vi "S2C_ExeScriptBreakPt.vi"(8 "Error In":errorcluster, 11 "Row":i32) -> (0 "Error Out":errorcluster)   [LabVIEW 2015]
doc: "Toggles the breakpoint symbol, for the selected line, on the executable script table"
uses:
  Globals/S2C_Globals.vi
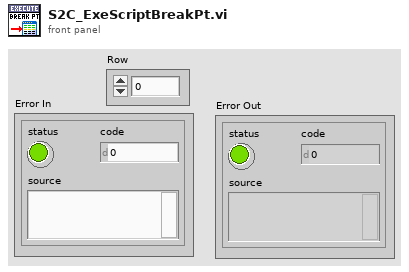
[diagram p1: front panel]
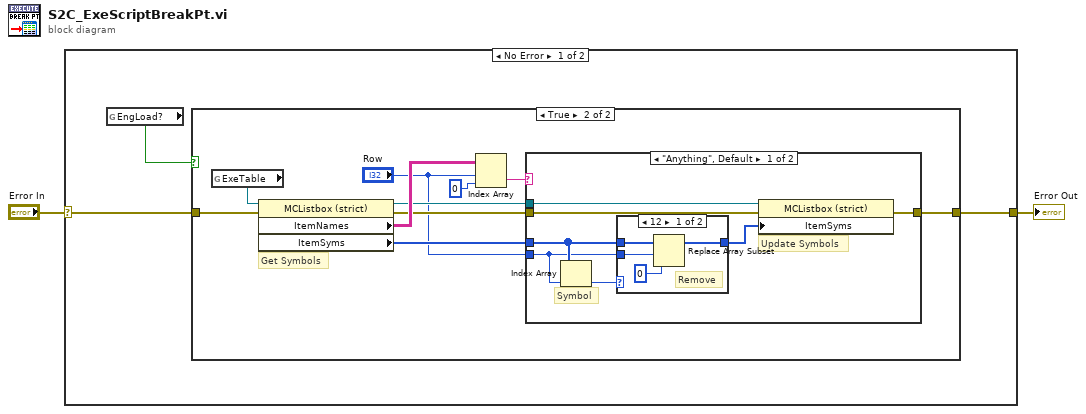
[diagram p0: block diagram]
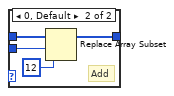
[diagram p3: hidden frame]
diagram:
  n1 = case shown="No Error" "Error In" {
    selector: "Error In" -> [w5 w33]
    tunnel: [w4 w33] -> w1
    frame No Error {
      n2 = global read "S2C_Globals.vi" "EngLoad?"() -> (w3:bool)
      n3 = case shown="True" w3 {
        tunnel: w5 -> [w6 w16]
        tunnel: [w6 w8] -> w4
        frame False {
          # "Breakpoints are only active for engineering loads"
        }
        frame True {
          # "Get Symbols"
          n4 = global read "S2C_Globals.vi" "ExeTable"() -> (w15:refnum<vi>)
          n5 = property class="MCListbox (strict)"(reference=w15, error in=w16) -> (reference out=w10:refnum<vi>, error out=w11:errorcluster, "ItemNames"=w14:string[][], "ItemSyms"=w9:i32[])
          n6 = Index Array(array=w14, index (row)="Row", index (col)=0 ("disabled index (col)")) -> (element=w12:string)
          n7 = case shown="\"Anything\", Default" w12 {
            tunnel: w11 -> [w20 w32]
            tunnel: w10 -> [w18 _]
            tunnel: w9 -> [w22 _]
            tunnel: [w17 w32] -> w8
            tunnel: "Row" -> [w21 _]
            frame "Anything", Default {
              # "Symbol"
              # "Update Symbols"
              n8 = Index Array(array=w22, index=w21) -> (element=w23:i32)
              n9 = case shown="12" w23 {
                tunnel: w22 -> [w27 w31]
                tunnel: w21 -> [w26 w30]
                tunnel: [w24 w28] -> w19
                frame 12 {
                  # "Remove"
                  n10 = Replace Array Subset(array=w27, new element=0, index=w26) -> (w24:i32[])
                }
                frame 0, Default {
                  # "Add"
                  n11 = Replace Array Subset(array=w31, new element=12, index=w30) -> (w28:i32[])
                }
              }
              n12 = property class="MCListbox (strict)"(reference=w18, error in=w20, "ItemSyms"=w19) -> (error out=w17:errorcluster)  [unwired: 1 out]
            }
            frame "" {
              # "Ignore if row blank"
            }
          }
        }
      }
    }
    frame Error {
    }
  }
  "Error Out" <- w1
